vi "convert_zerncoeffs.vi"(7 "ConType":T1(ring)=enum."Wyant2Wyant", 8 "error in (no error)":errorcluster, 10 "Zern coef in":dbl[](array[numeric])=[0.3, 0.0], 11 "Zern indx in":i32[](array[numeric])=[3, 4, 0, 0, 0, 0, 0, 0, 0, 0]) -> (0 "error out":errorcluster, 2 "Zern Coef Out":dbl[](array[numeric]), 3 "Zern index out":i32[](array[numeric])=[1, 2, 3, 4, 5, 6, 7, 8, 9, 8, 11, 12, 13, 14, 15, 16, 17, 18, 19, 20, 21, 22, 23, 24, 25, 26, 27, 28, 29, 30, 31, 32] min=1 max=32)   [LabVIEW 2018]
uses:
  <vilib>/Analysis/1siggen.llb/Ramp Pattern by Delta.vi
  <vilib>/Analysis/NI_AALBase.lvlib
panel:
  # "Convert zernike coefficients to extented coefficients with contineously squential indices\n0. ANSI2Wyant: ANSI convention to Wyant convention (50 indices output)\n1. Wyant2ANSI: Wyant convention to ANSI convention (35 indices output)\n2. ANSI2ANSI: ANSI convention to ANSI convention (35 indices output)\n3. Wyant2Wyant: Wyant convention to Wyant convention (50 indices output)"
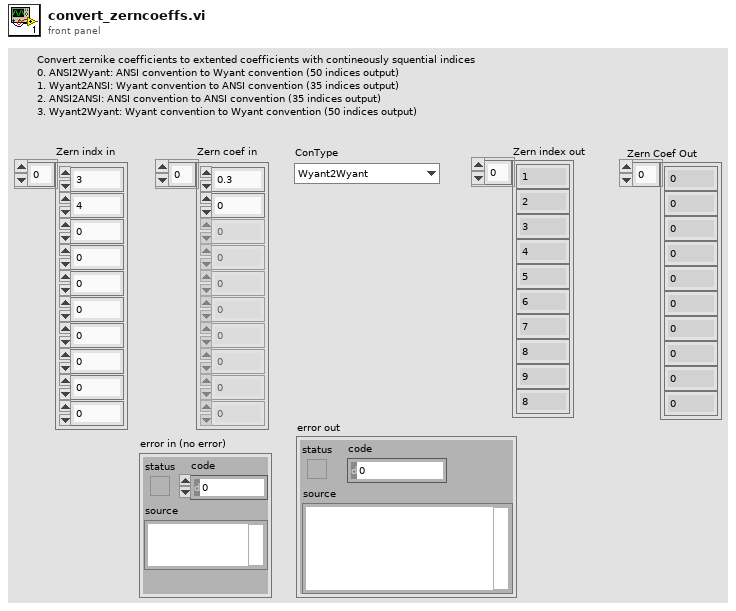
[diagram p1: front panel]
types:
  T1 = enum16{"ANSI2Wyant", "Wyant2ANSI", "ANSI2ANSI", "Wyant2Wyant"}
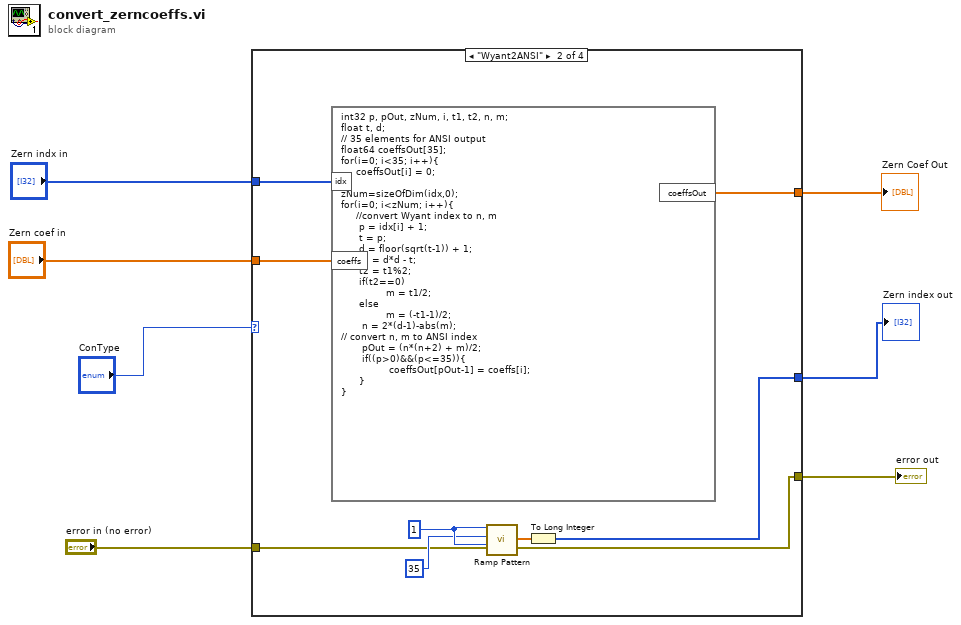
[diagram p0: block diagram]
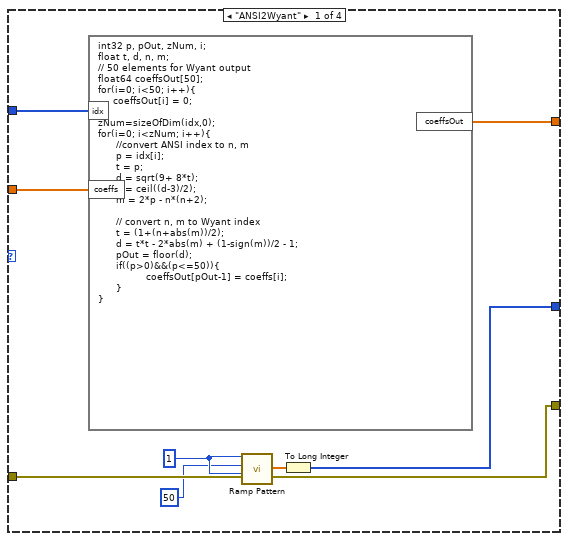
[diagram p2: hidden frame]
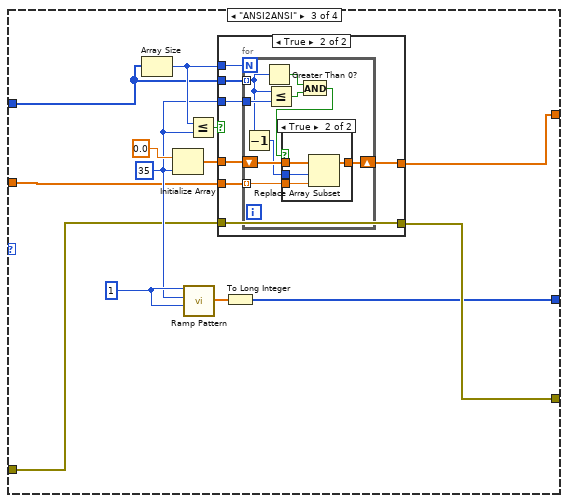
[diagram p3: hidden frame]
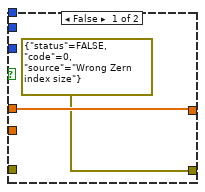
[diagram p4: hidden frame]
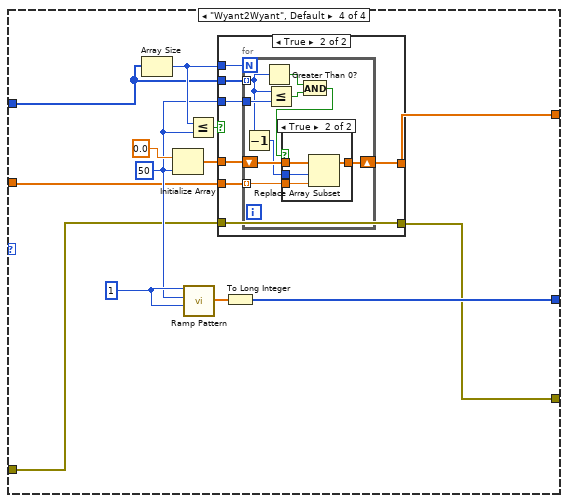
[diagram p6: hidden frame]
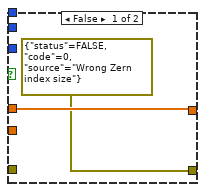
[diagram p7: hidden frame]
diagram:
  n1 = case shown="\"Wyant2ANSI\"" "ConType" {
    tunnel: "Zern coef in" -> [w15 w22 w28 w65]
    tunnel: [w14 w21 w24 w60] -> w6
    tunnel: "Zern indx in" -> [w13 w23 w27 w64]
    tunnel: [w9 w17 w25 w63] -> w3
    tunnel: [w12 w16 w26 w62] -> w2
    tunnel: "error in (no error)" -> [w12 w16 w29 w61]
    frame "ANSI2Wyant" {
      w11 = 1
      n2 = formula code="int32 p, pOut, zNum, i;\nfloat t, d, n, m;\n// 50 elements for Wyant output\nfloat64 coeffsOut[50];\nfor(i=0; i<50; i++){\n     coeffsOut[i] = 0;\n}\nzNum=sizeOfDim(idx,0);\nfor(i=0; i<zNum; i++){\n      //convert ANSI index to n, m\n      p = idx[i];\n      t = p;\n      d = sqrt(9+ 8*t);\n      n = ceil((d-3)/2);\n      m = 2*p - n*(n+2);\n\n      // convert n, m to Wyant index\n      t = (1+(n+abs(m))/2);\n      d = t*t - 2*abs(m) + (1-sign(m))/2 - 1;\n      pOut = floor(d);\n      if((p>0)&&(p<=50)){\n                coeffsOut[pOut-1] = coeffs[i];\n      }\n}"("coeffs"=w15, "idx"=w13) -> ("coeffsOut"=w14:dbl[])
      n3 = call-poly <vilib>:"Ramp Pattern.vi"("start"=w11, "end"=50, "delta"=w11) -> ("Ramp Pattern"=w10:dbl[])  [unwired: 6 in, 2 out]
      n4 = To Long Integer(number=w10) -> (32bit integer=w9:i32[])
    }
    frame "Wyant2ANSI" {
      w20 = 1
      n5 = formula code="int32 p, pOut, zNum, i, t1, t2, n, m;\nfloat t, d;\n// 35 elements for ANSI output\nfloat64 coeffsOut[35];\nfor(i=0; i<35; i++){\n     coeffsOut[i] = 0;\n}\nzNum=sizeOfDim(idx,0);\nfor(i=0; i<zNum; i++){\n     //convert Wyant index to n, m\n      p = idx[i] + 1;\n      t = p;\n      d = floor(sqrt(t-1)) + 1;\n      t1 = d*d - t;\n      t2 = t1%2;\n      if(t2==0)\n               m = t1/2;\n      else\n               m = (-t1-1)/2;\n       n = 2*(d-1)-abs(m);\n// convert n, m to ANSI index\n       pOut = (n*(n+2) + m)/2;\n       if((p>0)&&(p<=35)){\n                coeffsOut[pOut-1] = coeffs[i];\n      }\n}"("coeffs"=w22, "idx"=w23) -> ("coeffsOut"=w21:dbl[])
      n6 = call-poly <vilib>:"Ramp Pattern.vi"("start"=w20, "end"=35, "delta"=w20) -> ("Ramp Pattern"=w19:dbl[])  [unwired: 6 in, 2 out]
      n7 = To Long Integer(number=w19) -> (32bit integer=w17:i32[])
    }
    frame "ANSI2ANSI" {
      w35 = 1
      w30 = 35
      n8 = Array Size(array=w27) -> (size(s)=w31:i32)
      n9 = Initialize Array(0.0, w30) -> (w33:dbl[])
      n10 = call-poly <vilib>:"Ramp Pattern.vi"("start"=w35, "end"=w30, "delta"=w35) -> ("Ramp Pattern"=w34:dbl[])  [unwired: 6 in, 2 out]
      n11 = Less Or Equal?(x=w31, y=w30) -> (x <= y?=w32:bool)
      n12 = case shown="True" w32 {
        tunnel: w31 -> [_ w45]
        tunnel: w33 -> [w38 w44]
        tunnel: [w38 w43] -> w24
        tunnel: w27 -> [_ w42]
        tunnel: w28 -> [_ w41]
        tunnel: [errorcluster {"status"=FALSE, "code"=0, "source"="Wrong Zern index size"} ("error out") w40] -> w26
        tunnel: w29 -> [_ w40]
        tunnel: w30 -> [_ w39]
        frame False {
        }
        frame True {
          n13 = for {
            N: w45 -> [_]
            shift-right: [w53] -> w43
            shift-left: w44 -> [w54]
            tunnel: w42 -> [w49] mode=indexing
            tunnel: w41 -> [w52] mode=indexing
            tunnel: w39 -> [w50]
            n14 = Decrement(x=w49) -> (x-1=w51:i32)
            n15 = Greater Than 0?(x=w49) -> (x > 0?=w48:bool)
            n16 = Less Or Equal?(x=w49, y=w50) -> (x <= y?=w47:bool)
            n17 = And(x=w48, y=w47) -> (x .and. y?=w46:bool)
            n18 = case shown="True" w46 {
              tunnel: w51 -> [_ w59]
              tunnel: w54 -> [w55 w58]
              tunnel: [w55 w57] -> w53
              tunnel: w52 -> [_ w56]
              frame False {
              }
              frame True {
                n19 = Replace Array Subset(array=w58, new element=w56, index=w59) -> (w57:dbl[])
              }
            }
          }
        }
      }
      n20 = To Long Integer(number=w34) -> (32bit integer=w25:i32[])
    }
    frame "Wyant2Wyant", Default {
      w71 = 1
      w66 = 50
      n21 = Array Size(array=w64) -> (size(s)=w67:i32)
      n22 = Initialize Array(0.0, w66) -> (w69:dbl[])
      n23 = call-poly <vilib>:"Ramp Pattern.vi"("start"=w71, "end"=w66, "delta"=w71) -> ("Ramp Pattern"=w70:dbl[])  [unwired: 6 in, 2 out]
      n24 = Less Or Equal?(x=w67, y=w66) -> (x <= y?=w68:bool)
      n25 = case shown="True" w68 {
        tunnel: w67 -> [_ w81]
        tunnel: w69 -> [w74 w80]
        tunnel: [w74 w79] -> w60
        tunnel: w64 -> [_ w78]
        tunnel: w65 -> [_ w77]
        tunnel: [errorcluster {"status"=FALSE, "code"=0, "source"="Wrong Zern index size"} ("error out") w76] -> w62
        tunnel: w61 -> [_ w76]
        tunnel: w66 -> [_ w75]
        frame False {
        }
        frame True {
          n26 = for {
            N: w81 -> [_]
            shift-right: [w89] -> w79
            shift-left: w80 -> [w90]
            tunnel: w78 -> [w85] mode=indexing
            tunnel: w77 -> [w88] mode=indexing
            tunnel: w75 -> [w86]
            n27 = Decrement(x=w85) -> (x-1=w87:i32)
            n28 = Greater Than 0?(x=w85) -> (x > 0?=w84:bool)
            n29 = Less Or Equal?(x=w85, y=w86) -> (x <= y?=w83:bool)
            n30 = And(x=w84, y=w83) -> (x .and. y?=w82:bool)
            n31 = case shown="True" w82 {
              tunnel: w87 -> [_ w95]
              tunnel: w90 -> [w91 w94]
              tunnel: [w91 w93] -> w89
              tunnel: w88 -> [_ w92]
              frame False {
              }
              frame True {
                n32 = Replace Array Subset(array=w94, new element=w92, index=w95) -> (w93:dbl[])
              }
            }
          }
        }
      }
      n33 = To Long Integer(number=w70) -> (32bit integer=w63:i32[])
    }
  }
  "Zern Coef Out" <- w6
  "Zern index out" <- w3
  "error out" <- w2
